vi "Configure Trigger List.vi"(0 "VISA resource name":refnum<visa-resource-name>, 1 "Trigger Slope":i32(ring) items=["Positive", "Negative"], 5 "Trigger Delay List":dbl[](array[numeric])=[0.0, 0.0, 0.0], 7 "Trigger Level":dbl, 9 "Trigger Source":i32(ring) items=["External1", "External2", "Immediate", "BUS"], 11 "error in (no error)":errorcluster, 12 "Trigger Holdoff":dbl) -> (4 "VISA resource name out":refnum<visa-resource-name>, 15 "error out":errorcluster)   [LabVIEW 2018, in "Agilent MXA Series.lvlib"]
doc: "Cofigures the Trigger Settings under List Sweep measurement type."
uses:
  Agilent MXA Series.lvlib
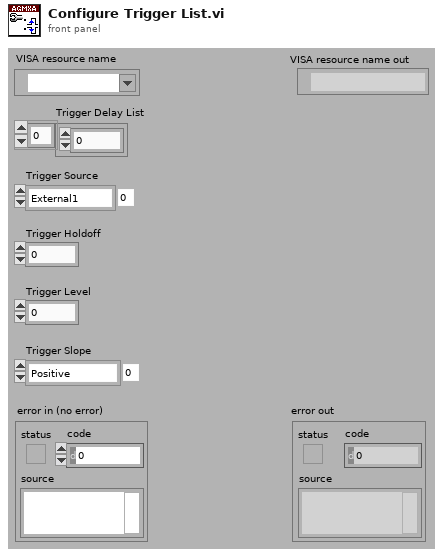
[diagram p1: front panel]
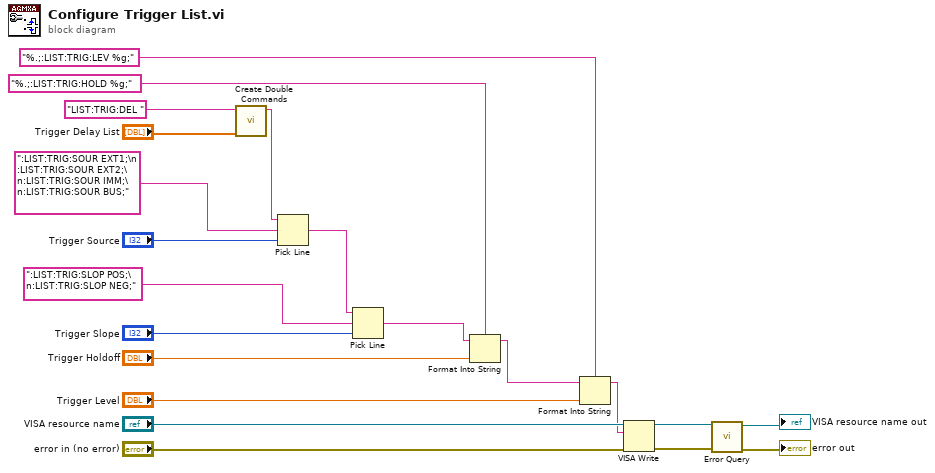
[diagram p0: block diagram]
diagram:
  n1 = call "Create Double Commands.vi"("Double Values"="Trigger Delay List", "Commands"="LIST:TRIG:DEL ") -> ("Result"=w2:string)  [unwired: 9 in]
  n2 = Pick Line(string ("")=w2, multi-line string=":LIST:TRIG:SOUR EXT1;\n :LIST:TRIG:SOUR EXT2;\n:LIST:TRIG:SOUR IMM;\n:LIST:TRIG:SOUR BUS;", line index="Trigger Source") -> (output string=w7:string)
  n3 = Pick Line(string ("")=w7, multi-line string=":LIST:TRIG:SLOP POS;\n:LIST:TRIG:SLOP NEG;", line index="Trigger Slope") -> (output string=w4:string)
  n4 = Format Into String(format string="%.;:LIST:TRIG:HOLD %g;", initial string=w4, "Trigger Holdoff") -> (resulting string=w3:string)  [unwired: 1 in, 1 out]
  n5 = Format Into String(format string="%.;:LIST:TRIG:LEV %g;", initial string=w3, "Trigger Level") -> (resulting string=w1:string)  [unwired: 1 in, 1 out]
  n6 = VISA Write(VISA resource name="VISA resource name", write buffer=w1, error in (no error)="error in (no error)") -> (VISA resource name out=w12:refnum<visa-resource-name>, error out=w13:errorcluster)  [unwired: 1 out]
  n7 = call "Error Query.vi"("error in (no error)"=w13, "VISA resource name"=w12) -> ("error out"=→"error out":errorcluster, "VISA resource name out"=→"VISA resource name out":refnum<visa-resource-name>)  [unwired: 6 in, 2 out]
